vi "IO_txt_writer.vi"(0 "info_sheet":string, 1 "path":path, 2 "y_data_arr":dbl[][](array[numeric]), 3 "x_data_arr":dbl[][](array[numeric])) -> ()   [LabVIEW 2014]
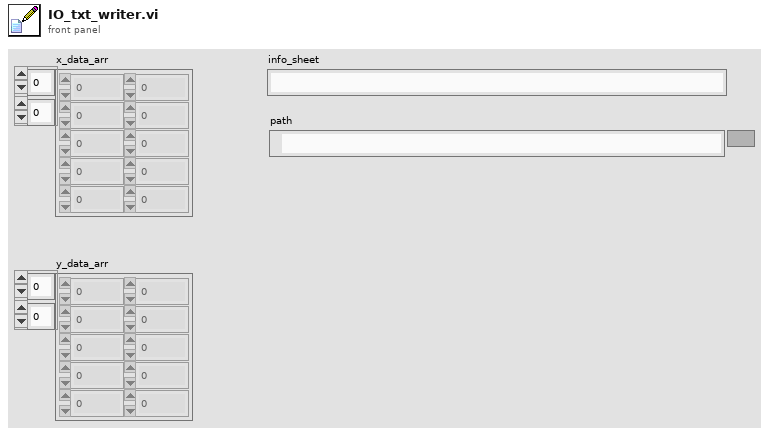
[diagram p1: front panel]
types:
  T1 = enum16{"open", "replace", "create", "open or create", "replace or create", "replace or create with confirmation"}
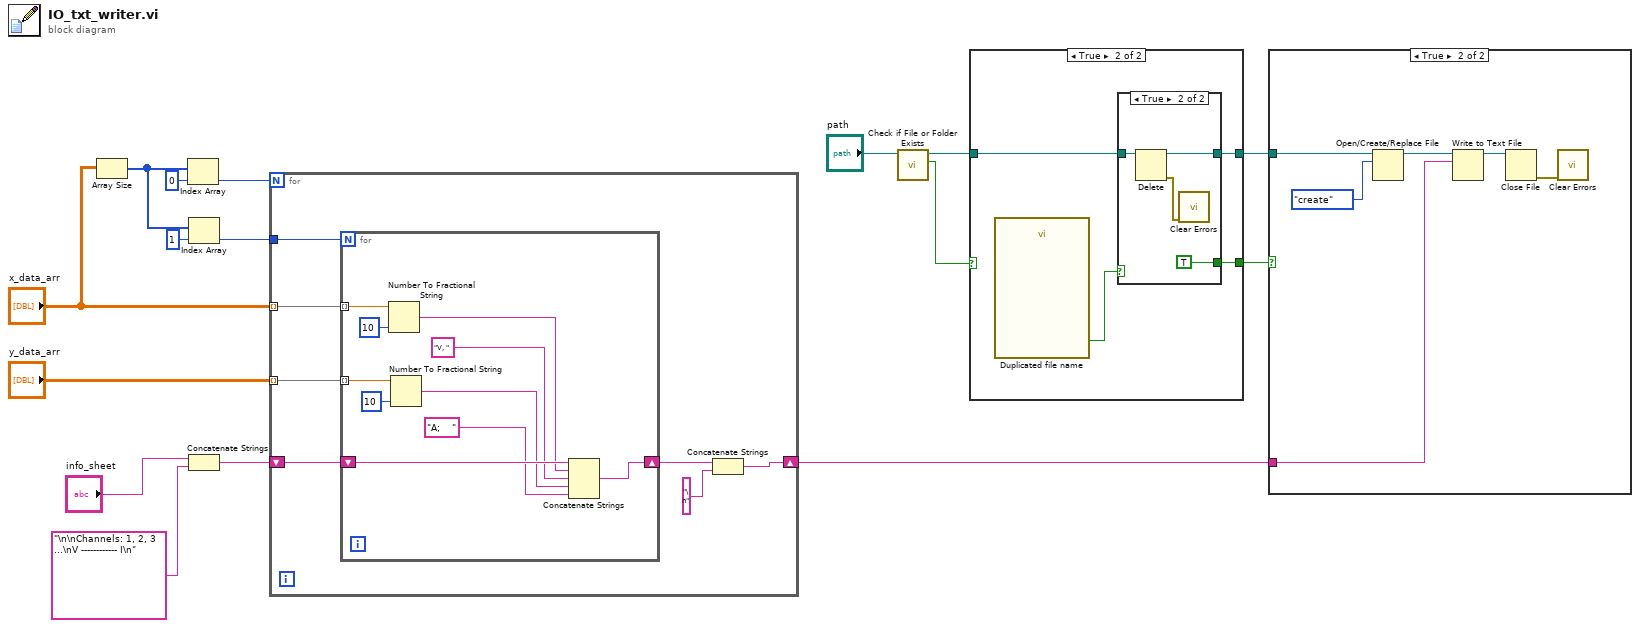
[diagram p0: block diagram]
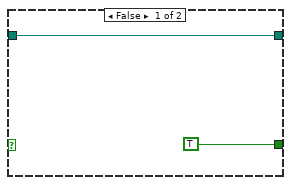
[diagram p3: hidden frame]
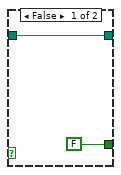
[diagram p4: hidden frame]
diagram:
  n1 = Array Size(array="x_data_arr") -> (size(s)=w10:i32[])
  n2 = Index Array(array=w10, index=0) -> (element=w12:i32)
  n3 = Index Array(array=w10, index=1) -> (element=w9:i32)
  n4 = Concatenate Strings("info_sheet", "\n\nChannels: 1, 2, 3 ...\nV ------------ I\n" ("string")) -> (w7:string)
  n5 = for {
    N: w12 -> [_]
    tunnel: "x_data_arr" -> [w22] mode=indexing
    tunnel: w9 -> [w23]
    tunnel: "y_data_arr" -> [w21] mode=indexing
    shift-right: [w18] -> w1
    shift-left: w7 -> [w20]
    n6 = for {
      N: w23 -> [_]
      tunnel: w22 -> [w33] mode=indexing
      tunnel: w21 -> [w30] mode=indexing
      shift-right: [w24] -> w19
      shift-left: w20 -> [w29]
      n7 = Number To Fractional String(number=w33, precision (6)=i16 10) -> (F-format string=w28:string)  [unwired: 2 in]
      n8 = Number To Fractional String(number=w30, precision (6)=i16 10) -> (F-format string=w26:string)  [unwired: 2 in]
      n9 = Concatenate Strings(w29, w28, "V, " ("string"), w26, "A;    " ("string")) -> (w24:string)
    }
    n10 = Concatenate Strings(w19, "\n" ("string")) -> (w18:string)
  }
  n11 = call <vilib>:"Check if File or Folder Exists.vi"("path"="path") -> ("file or folder exists?"=w5:bool, "dup path"=w4:path)  [unwired: 8 in, 1 out]
  n12 = case shown="True" w5 {
    tunnel: w4 -> [w34 w38]
    tunnel: [TRUE w37] -> w3
    tunnel: [w34 w36] -> w2
    frame False {
    }
    frame True {
      n13 = call "Duplicated file name"() -> ("OK"=w39:bool)  [unwired: 10 in, 1 out]
      n14 = case shown="True" w39 {
        tunnel: w38 -> [w40 w44]
        tunnel: [FALSE TRUE] -> w37
        tunnel: [w40 w43] -> w36
        frame False {
        }
        frame True {
          n15 = Delete(path (use dialog)=w44) -> (deleted path=w43:path, error out=w42:errorcluster)  [unwired: 4 in, 1 out]
          n16 = call <vilib>:"Clear Errors.vi"("error in (no error)"=w42) -> ()  [unwired: 5 in, 2 out]
        }
      }
    }
  }
  n17 = case shown="True" w3 {
    tunnel: w2 -> [_ w50]
    tunnel: w1 -> [_ w48]
    frame False {
    }
    frame True {
      n18 = Open/Create/Replace File(file path (use dialog)=w50, operation (0:open)=T1."create") -> (refnum out=w49:refnum<file>)  [unwired: 4 in, 2 out]
      n19 = Write to Text File(file (use dialog)=w49, text=w48) -> (refnum out=w47:refnum<file>)  [unwired: 2 in, 2 out]
      n20 = Close File(refnum=w47) -> (error out=w46:errorcluster)  [unwired: 1 in, 1 out]
      n21 = call <vilib>:"Clear Errors.vi"("error in (no error)"=w46) -> ()  [unwired: 5 in, 2 out]
    }
  }
